vi "Read_register _values_1.vi"(8 "error in":errorcluster) -> (0 "error out":errorcluster, 3 "Data":u8)   [LabVIEW 2018]
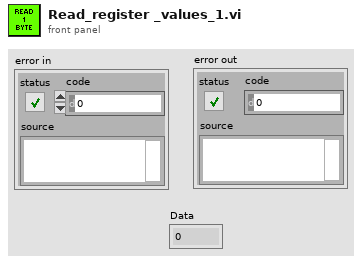
[diagram p1: front panel]
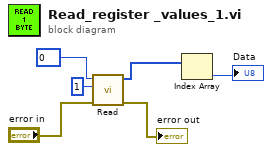
[diagram p0: block diagram]
diagram:
  n1 = call "Read.vi"("error in"="error in", "Byte Count"=u32 1, "Byte to Write"=u8 0 ("Slave Address (7-bit)")) -> ("error out"=→"error out":errorcluster, "Bytes Read"=w3:u8[])  [unwired: 7 in]
  n2 = Index Array(array=w3) -> (element=→"Data":u8)  [unwired: 1 in]
